vi "Find Generic Data Frame Sync Bytes over TCP.vi"(8 "error in (no error)":errorcluster, 11 "TCP Network Connection in":refnum<k5>) -> (0 "error out":errorcluster, 2 "Valid Sync":bool, 3 "TCP Network Connection out":refnum<k5>)   [LabVIEW 2023]
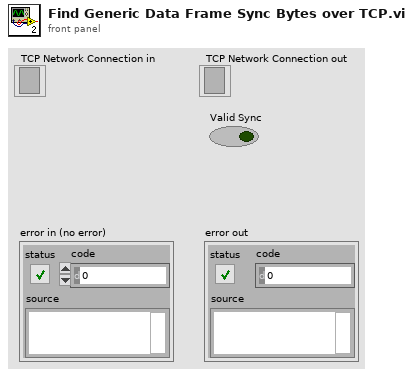
[diagram p1: front panel]
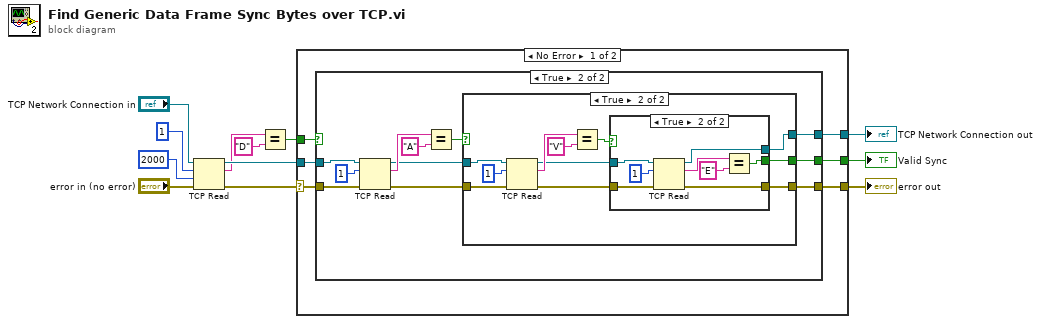
[diagram p0: block diagram]
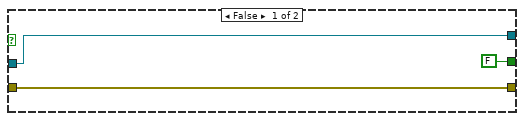
[diagram p2: hidden frame]
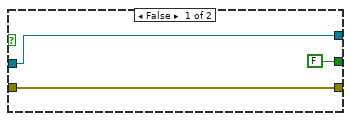
[diagram p3: hidden frame]
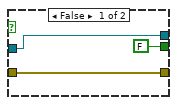
[diagram p4: hidden frame]
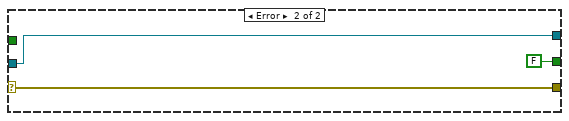
[diagram p5: hidden frame]
diagram:
  n1 = TCP Read(connection ID="TCP Network Connection in", bytes to read=1, error in (no error)="error in (no error)", 9:2000 ("timeout ms (25000)")) -> (connection ID out=w9:refnum<k5>, data out=w6:string, error out=w1:errorcluster)  [unwired: 1 in]
  n2 = Equal?(x=w6, y="D") -> (x = y?=w8:bool)
  n3 = case shown="No Error" w1 {
    selector: w1 -> [w13 w60]
    tunnel: [w18 w60] -> w12
    tunnel: [w17 w59] -> w11
    tunnel: [w16 FALSE] -> w10
    tunnel: w9 -> [w15 w59]
    tunnel: w8 -> [w14 _]
    frame No Error {
      n4 = case shown="True" w14 {
        tunnel: w15 -> [w19 w31]
        tunnel: [FALSE w26] -> w16
        tunnel: [w19 w25] -> w17
        tunnel: w13 -> [w20 w24]
        tunnel: [w20 w22] -> w18
        frame False {
        }
        frame True {
          n5 = TCP Read(connection ID=w31, bytes to read=1, error in (no error)=w24) -> (connection ID out=w27:refnum<k5>, data out=w30:string, error out=w23:errorcluster)  [unwired: 2 in]
          n6 = Equal?(x=w30, y="A") -> (x = y?=w28:bool)
          n7 = case shown="True" w28 {
            tunnel: w27 -> [w34 w43]
            tunnel: [FALSE w40] -> w26
            tunnel: [w34 w39] -> w25
            tunnel: w23 -> [w33 w38]
            tunnel: [w33 w36] -> w22
            frame False {
            }
            frame True {
              n8 = TCP Read(connection ID=w43, bytes to read=1, error in (no error)=w38) -> (connection ID out=w41:refnum<k5>, data out=w45:string, error out=w37:errorcluster)  [unwired: 2 in]
              n9 = Equal?(x=w45, y="V") -> (x = y?=w42:bool)
              n10 = case shown="True" w42 {
                tunnel: w41 -> [w47 w56]
                tunnel: [FALSE w53] -> w40
                tunnel: [w47 w52] -> w39
                tunnel: w37 -> [w48 w51]
                tunnel: [w48 w50] -> w36
                frame False {
                }
                frame True {
                  n11 = TCP Read(connection ID=w56, bytes to read=1, error in (no error)=w51) -> (connection ID out=w52:refnum<k5>, data out=w54:string, error out=w50:errorcluster)  [unwired: 2 in]
                  n12 = Equal?(x=w54, y="E") -> (x = y?=w53:bool)
                }
              }
            }
          }
        }
      }
    }
    frame Error {
    }
  }
  "error out" <- w12
  "TCP Network Connection out" <- w11
  "Valid Sync" <- w10
